vi "commit.vi"(8 "error in":errorcluster, 9 "Timeout (ms)":i32=-1, 11 "profibus reference":T1) -> (0 "error out":errorcluster, 3 "profibus reference out":T1)   [LabVIEW 2013, in "dynamic profibus.lvlib"]
uses:
  dynamic profibus.lvlib
  fpga reference.ctl
  profibus master action.ctl
  <vilib>/rvi/interface/common/niFpgaWaitOnOcc.vi
  <vilib>/Utility/error.llb/Error Cluster From Error Code.vi
  <vilib>/rvi/errors/niLvFpgaAdjustHostInterfaceError.vi
  <vilib>/rvi/interface/nirviMethod/nirviMethod.xnode
  <vilib>/FPGAPlugInAG/Dynamic/niLvFpga_WriteFifo_Dynamic.vi
  <vilib>/rvi/errors/niLvFpgaMergeErrorWithErrorCode.vi
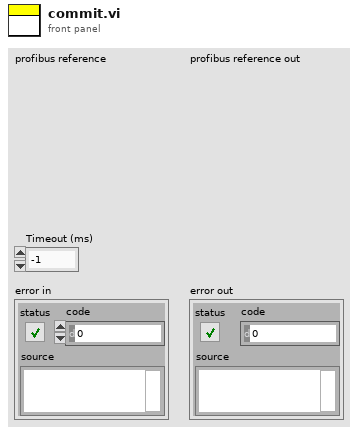
[diagram p1: front panel]
types:
  T1 = typedef "dynamic profibus.lvlib/fpga reference.ctl" = refnum<k20>
  T2 = typedef "profibus master action.ctl" = enum8{"set output", "transfer complete", "configure reads", "configure diagnostics"}
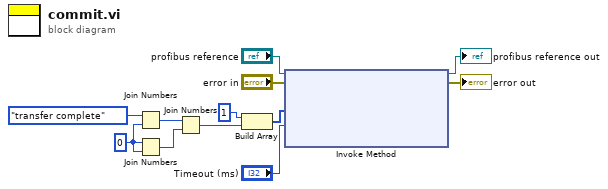
[diagram p0: block diagram]
diagram:
  w2 = u8 0 ("lo")
  n1 = Join Numbers(hi=profibus_master_action."transfer complete" ("action"), lo=w2) -> ((hi.lo)=w4:u16)
  n2 = Join Numbers(hi=w2, lo=w2) -> ((hi.lo)=w3:u16)
  n3 = Join Numbers(hi=w4, lo=w3) -> ((hi.lo)=w1:u32)
  n4 = Build Array(u32 1, w1) -> (w7:u32[])
  n5 = xnode "Invoke Method"("FPGA VI Reference In"="profibus reference", "error in"="error in", "Data"=w7, "Timeout (ms)"="Timeout (ms)") -> ("FPGA VI Reference Out"=→"profibus reference out":T1, "error out"=→"error out":errorcluster)  [unwired: 1 out]
